vi "Configure Digital Trigger Output Line.vi"(6 "Stimulus Event":u16(ring) items=["None", "Front Pannel Trigger Key", "Notify Trigger Block 1", "Notify Trigger Block 2", "Notify Trigger Block 3", "Notify Trigger Block 4", "Notify Trigger Block 5", "Notify Trigger Block 6", "Notify Trigger Block 7", "Notify Trigger Block 8", "Command", "Digi IO Line 1", "Digi IO Line 2", "Digi IO Line 3", "Digi IO Line 4", "Digi IO Line 5", "Digi IO Line 6", "TSP-Link 1", "TSP-Link 2", "TSP-Link 3", "LAN 1", "LAN 2", "LAN 3", "LAN 4", "LAN 5", "LAN 6", "LAN 7", "LAN 8", "Blender 1", "Blender 2", "Timer 1", "Timer 2", "Timer 3", "Timer 4", "Analog Trigger", "External Trigger"], 8 "error in (no error)":errorcluster, 9 "Trigger Logic Type":u16(ring) items=["Positive", "Negative"], 10 "Digital IO Line (1)":u32=1 min=1 max=6 step=1, 11 "VISA resource name":refnum<visa-resource-name>) -> (0 "error out":errorcluster, 3 "VISA resource name out":refnum<visa-resource-name>)   [LabVIEW 2018, in "Keithley DMM7512.lvlib"]
doc: "This VI sets the output logic of the trigger event generator, pulse width and output stimulus."
uses:
  <instrlib>/Keithley DMM7512/Keithley DMM7512.lvlib
panel:
  in  "Pulse width (10 us)":dbl=1e-05
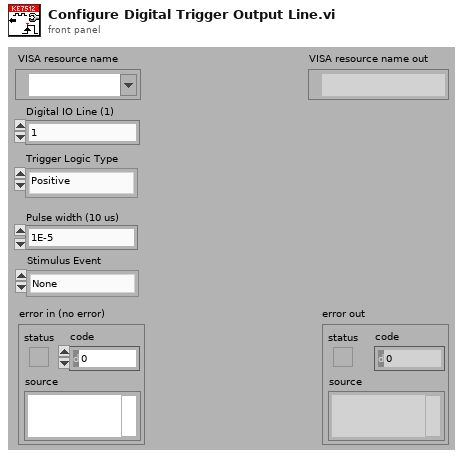
[diagram p1: front panel]
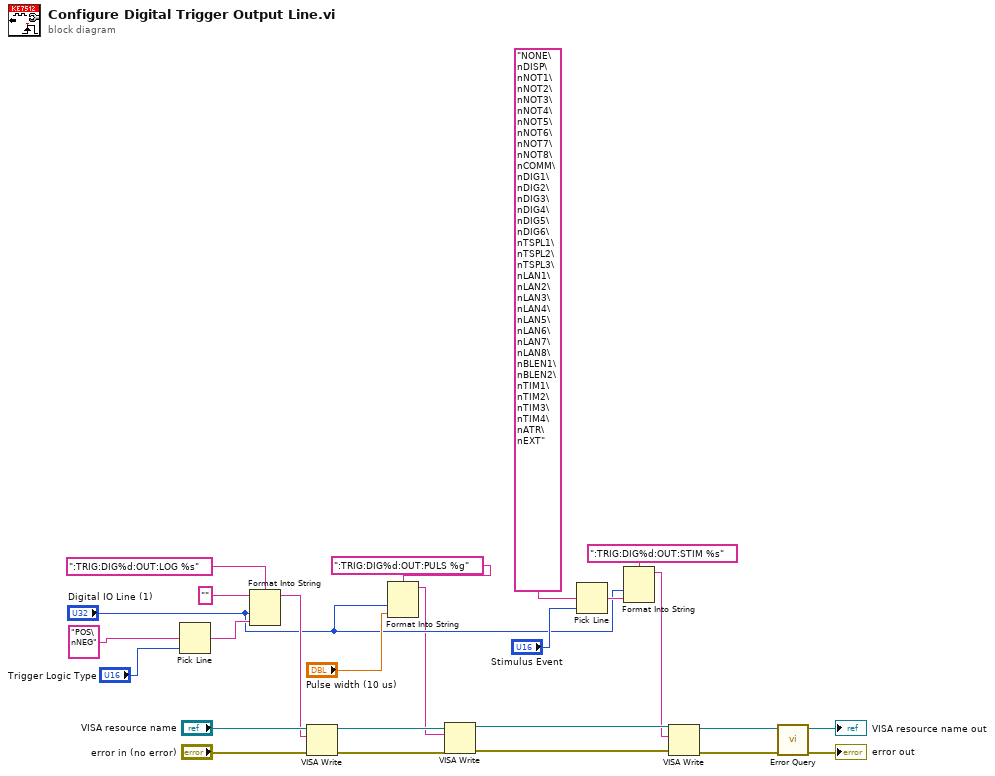
[diagram p0: block diagram]
diagram:
  n1 = Pick Line(multi-line string="POS\nNEG", line index="Trigger Logic Type") -> (output string=w16:string)  [unwired: 1 in]
  n2 = Format Into String(format string=":TRIG:DIG%d:OUT:LOG %s", initial string="", "Digital IO Line (1)", w16) -> (resulting string=w19:string)  [unwired: 1 in, 1 out]
  n3 = VISA Write(VISA resource name="VISA resource name", write buffer=w19, error in (no error)="error in (no error)") -> (VISA resource name out=w9:refnum<visa-resource-name>, error out=w8:errorcluster)  [unwired: 1 out]
  n4 = Format Into String(format string=":TRIG:DIG%d:OUT:PULS %g", "Digital IO Line (1)", "Pulse width (10 us)") -> (resulting string=w7:string)  [unwired: 2 in, 1 out]
  n5 = VISA Write(VISA resource name=w9, write buffer=w7, error in (no error)=w8) -> (VISA resource name out=w5:refnum<visa-resource-name>, error out=w4:errorcluster)  [unwired: 1 out]
  n6 = Pick Line(multi-line string="NONE\nDISP\nNOT1\nNOT2\nNOT3\nNOT4\nNOT5\nNOT6\nNOT7\nNOT8\nCOMM\nDIG1\nDIG2\nDIG3\nDIG4\nDIG5\nDIG6\nTSPL1\nTSPL2\nTSPL3\nLAN1\nLAN2\nLAN3\nLAN4\nLAN5\nLAN6\nLAN7\nLAN8\nBLEN1\nBLEN2\nTIM1\nTIM2\nTIM3\nTIM4\nATR\nEXT", line index="Stimulus Event") -> (output string=w12:string)  [unwired: 1 in]
  n7 = Format Into String(format string=":TRIG:DIG%d:OUT:STIM %s", "Digital IO Line (1)", w12) -> (resulting string=w1:string)  [unwired: 2 in, 1 out]
  n8 = VISA Write(VISA resource name=w5, write buffer=w1, error in (no error)=w4) -> (VISA resource name out=w2:refnum<visa-resource-name>, error out=w3:errorcluster)  [unwired: 1 out]
  n9 = call <instrlib>:"Error Query.vi"("error in (no error)"=w3, "VISA resource name"=w2) -> ("error out"=→"error out":errorcluster, "VISA resource name out"=→"VISA resource name out":refnum<visa-resource-name>)  [unwired: 8 out]
